vi "HEWH_HeiseBarometer.vi"(8 "error in":errorcluster, 11 "Message Queues out":T1) -> (0 "error out":errorcluster)   [LabVIEW 2023]
uses:
  Tenney/support/Message Queue/All Message Queues.ctl
  Tenney/support/Message Queue/Message Cluster.ctl
  FVIR and LDO/support/Message Queue/Enqueue Message (Single).vi
  FVIR and LDO/support/Message Queue/Message Queue.lvlib
  Tenney/support/Message Queue/Tenney Message Queue.lvlib
panel:
  out "Barometric Pressure (in Hg)":dbl
  out "Debug":string[](array[string])
  in  "Debug":bool
  out "Loop Count":i32
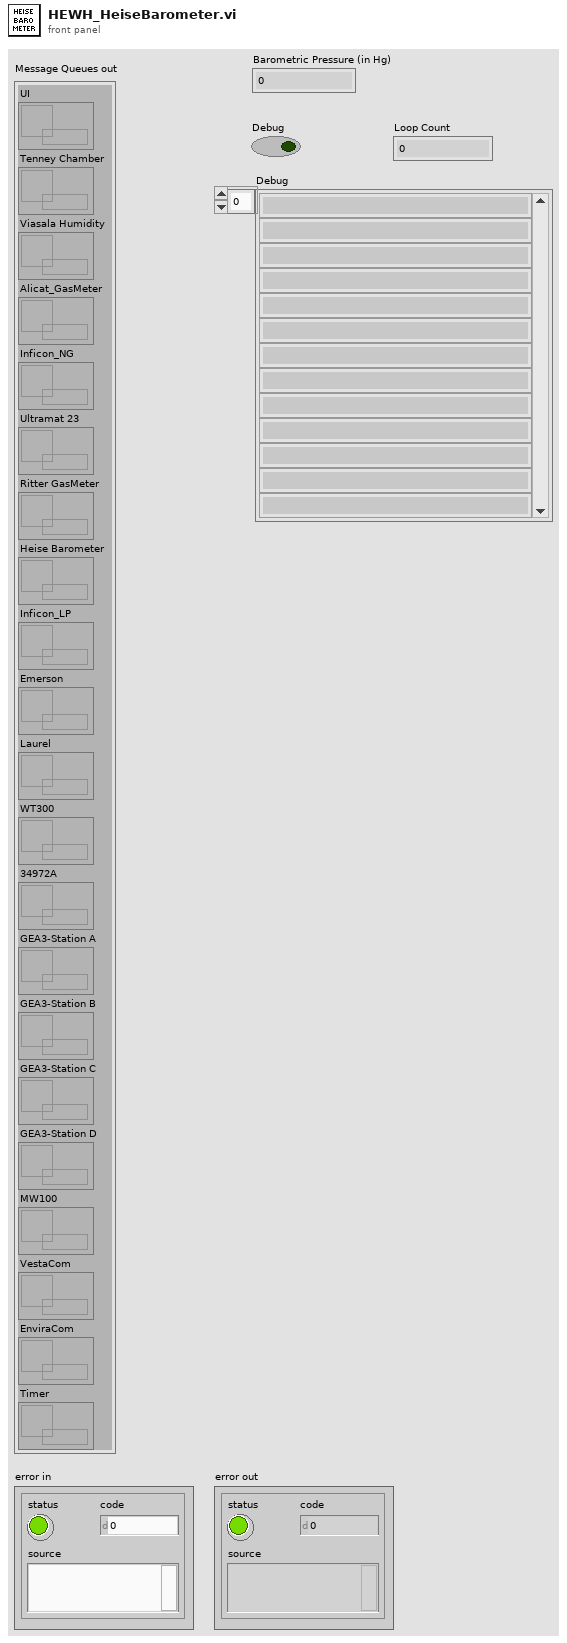
[diagram p1: front panel]
types:
  T1 = typedef "Tenney Message Queue.lvlib/All Message Queues.ctl" = cluster{"UI":refnum<queue>, "Tenney Chamber":refnum<queue>, "Viasala Humidity":refnum<queue>, "Alicat_GasMeter":refnum<queue>, "Inficon_NG":refnum<queue>, "Ultramat 23":refnum<queue>, "Ritter GasMeter":refnum<queue>, "Heise Barometer":refnum<queue>, "Inficon_LP":refnum<queue>, "Emerson":refnum<queue>, "Laurel":refnum<queue>, "WT300":refnum<queue>, "34972A":refnum<queue>, "GEA3-Station A":refnum<queue>, "GEA3-Station B":refnum<queue>, "GEA3-Station C":refnum<queue>, "GEA3-Station D":refnum<queue>, "MW100":refnum<queue>, "VestaCom":refnum<queue>, "EnviraCom":refnum<queue>, "Timer":refnum<queue>}
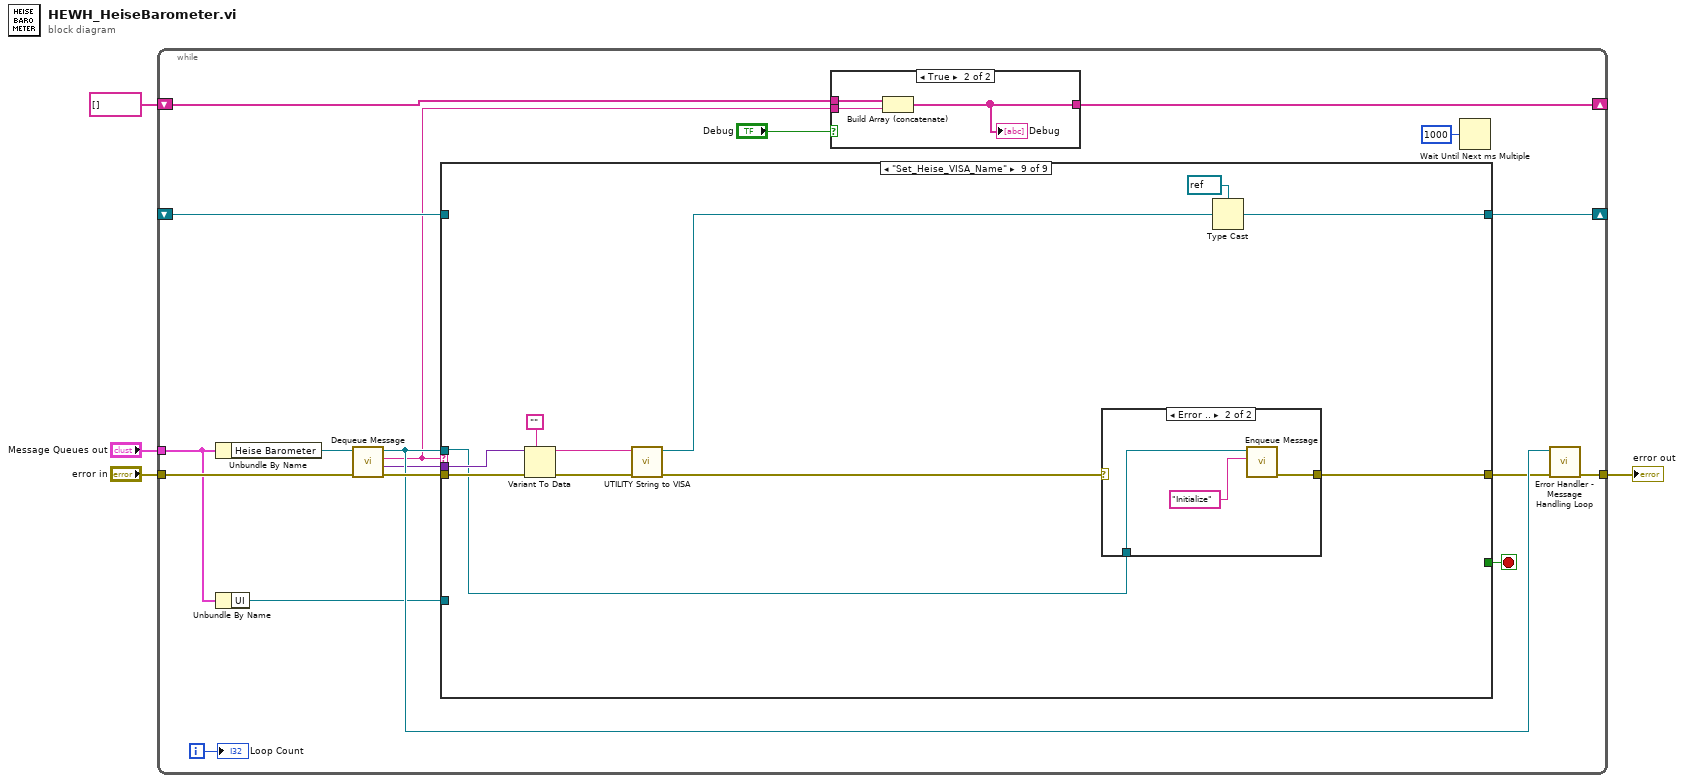
[diagram p0: block diagram]
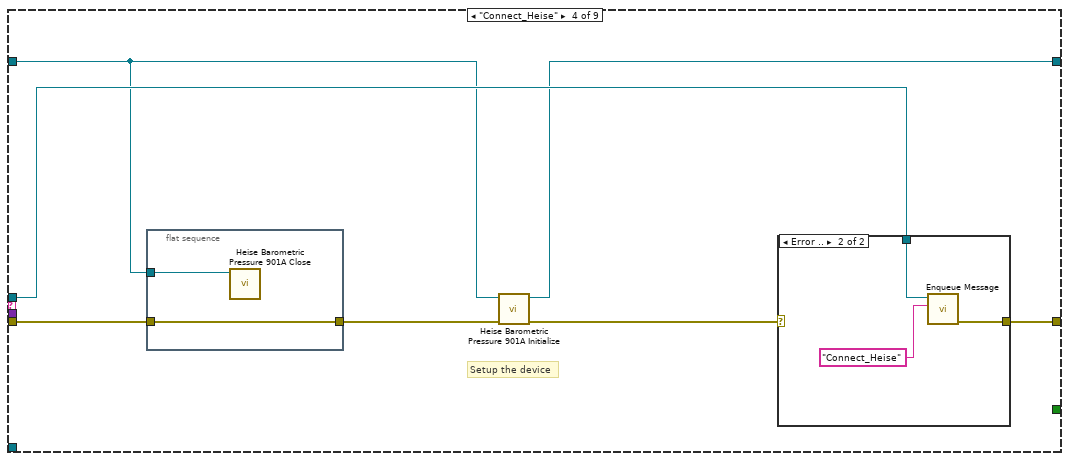
[diagram p6: hidden frame]
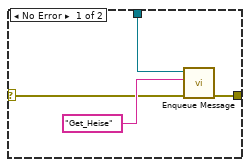
[diagram p7: hidden frame]
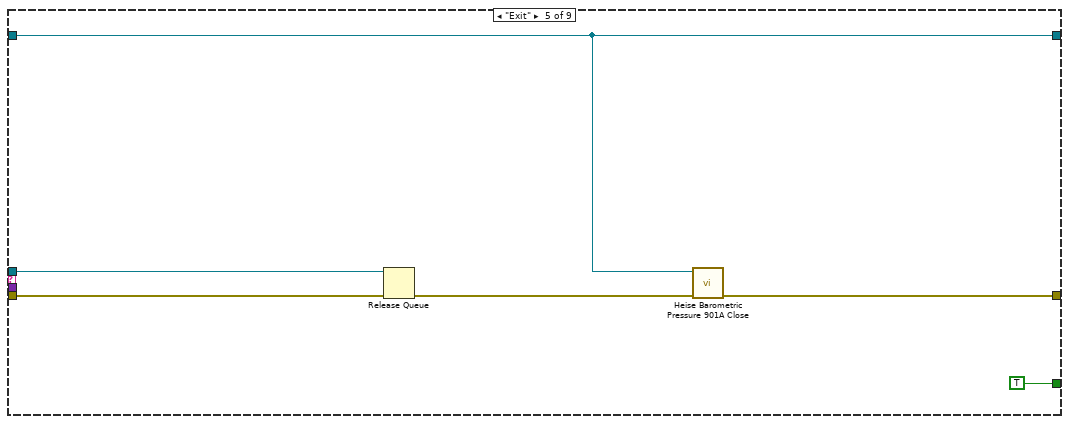
[diagram p8: hidden frame]
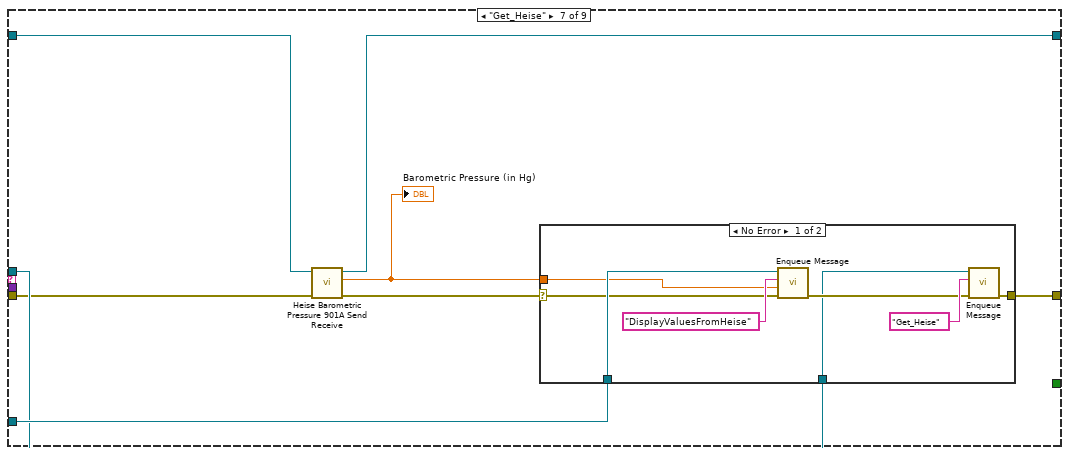
[diagram p10: hidden frame]
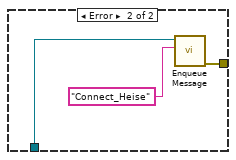
[diagram p11: hidden frame]
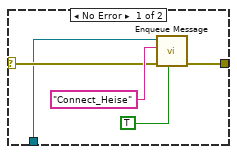
[diagram p13: hidden frame]
diagram:
  n1 = while {
    tunnel: "Message Queues out" -> [w14]
    tunnel: "error in" -> [w21]
    tunnel: [w17] -> w3
    shift-right: [w12] -> _
    shift-left: _ -> [w11]
    shift-right: [w6] -> _
    shift-left: string[] [] -> [w8]
    i -> [w10]
    stop <- w19 stop-if-true
    n2 = Unbundle By Name(w14) -> ("Heise Barometer"=w22:refnum<queue>)
    n3 = Unbundle By Name(w14) -> ("UI"=w13:refnum<queue>)
    n4 = call "Dequeue Message.vi"("error in (no error)"=w21, "Message Queue"=w22) -> ("error out"=w20:errorcluster, "Message Data"=w5:variant, "Message"=w7:string, "dup Message Queue"=w18:refnum<queue>)  [unwired: 6 in]
    n5 = case shown="\"Set_Heise_VISA_Name\"" w7 {
      tunnel: w20 -> [w27 w29 w31 w35 w49 w55 w61 w76 w87]
      tunnel: [w27 w29 w31 w39 w51 w55 w63 w76 w82] -> w16
      tunnel: [_ _ _ _ TRUE _ _ _ _] -> w19
      tunnel: w18 -> [_ _ _ w38 w53 _ w62 _ w81]
      tunnel: w13 -> [_ _ _ _ _ _ w64 _ _]
      tunnel: [w28 w30 w32 w37 w50 w56 w59 w77 w78] -> w12
      tunnel: w11 -> [w28 w30 w32 w34 w50 w56 w60 w77 _]
      tunnel: w5 -> [_ _ _ _ _ _ _ _ w86]
      frame "---------- Setup ----------" {
      }
      frame Default {
      }
      frame "Initialize" {
      }
      frame "Connect_Heise" {
        # "Setup the device"
        n6 = flat-sequence {
          tunnel: w35 -> [w40]
          tunnel: w34 -> [w41]
          tunnel: [w40] -> w33
          frame #0 {
            n7 = call "Heise Barometric Pressure 901A Close.vi"("VISA Refnum in"=w41) -> ()  [unwired: 10 in, 1 out]
          }
        }
        n8 = call "Heise Barometric Pressure 901A Initialize.vi"("error in (no error)"=w33, "VISA Refnum in"=w34) -> ("error out"=w36:errorcluster, "VISA Refnum out"=w37:refnum<visa-resource-name>)  [unwired: 8 in]
        n9 = case shown="Error .." w36 {
          selector: w36 -> [w42 _]
          tunnel: [w44 w47] -> w39
          tunnel: w38 -> [w43 w46]
          frame No Error {
            n10 = call-poly "Enqueue Message.vi"("error in (no error)"=w42, "Message"="Get_Heise", "Message Queue"=w43) -> ("error out"=w44:errorcluster)  [unwired: 7 in, 1 out]
          }
          frame Error {
            n11 = call-poly "Enqueue Message.vi"("Message"="Connect_Heise", "Message Queue"=w46) -> ("error out"=w47:errorcluster)  [unwired: 8 in, 1 out]
          }
        }
      }
      frame "Exit" {
        n12 = Release Queue(queue=w53, error in (no error)=w49) -> (error out=w52:errorcluster)  [unwired: 1 in, 2 out]
        n13 = call "Heise Barometric Pressure 901A Close.vi"("error in (no error)"=w52, "VISA Refnum in"=w50) -> ("error out"=w51:errorcluster)  [unwired: 9 in]
      }
      frame "---------- Data Collection ----------" {
      }
      frame "Get_Heise" {
        n14 = call "Heise Barometric Pressure 901A Send Receive.vi"("error in (no error)"=w61, "VISA Refnum in"=w60) -> ("error out"=w57:errorcluster, "Barometric Pressure (in Hg)"=w58:dbl, "VISA Refnum out"=w59:refnum<visa-resource-name>)  [unwired: 5 in, 2 out]
        "Barometric Pressure (in Hg)" <- w58
        n15 = case shown="No Error" w57 {
          selector: w57 -> [w65 _]
          tunnel: w64 -> [w71 _]
          tunnel: [w68 w74] -> w63
          tunnel: w62 -> [w67 w73]
          tunnel: w58 -> [w66 _]
          frame No Error {
            n16 = call-poly "Enqueue Message.vi"("error in (no error)"=w65, "Message Data"=w66, "Message"="DisplayValuesFromHeise", "Message Queue"=w71) -> ("error out"=w69:errorcluster)  [unwired: 6 in, 1 out]
            n17 = call-poly "Enqueue Message.vi"("error in (no error)"=w69, "Message"="Get_Heise", "Message Queue"=w67) -> ("error out"=w68:errorcluster)  [unwired: 7 in, 1 out]
          }
          frame Error {
            n18 = call-poly "Enqueue Message.vi"("Message"="Connect_Heise", "Message Queue"=w73) -> ("error out"=w74:errorcluster)  [unwired: 8 in, 1 out]
          }
        }
      }
      frame "---------- Events ----------" {
      }
      frame "Set_Heise_VISA_Name" {
        n19 = Variant To Data(error in=w87, type="", Variant=w86) -> (data=w84:string, error out=w85:errorcluster)
        n20 = call "UTILITY String to VISA.vi"("error in (no error)"=w85, "VISA Name"=w84) -> ("error out"=w83:errorcluster, "VISA resource name out"=w80:refnum<visa-resource-name>)  [unwired: 8 in]
        n21 = case shown="Error .." w83 {
          selector: w83 -> [w91 _]
          tunnel: [w90 w95] -> w82
          tunnel: w81 -> [w89 w94]
          frame No Error {
            n22 = call-poly "Enqueue Message.vi"("Priority Message? (F)"=TRUE, "error in (no error)"=w91, "Message"="Connect_Heise", "Message Queue"=w89) -> ("error out"=w90:errorcluster)  [unwired: 6 in, 1 out]
          }
          frame Error {
            n23 = call-poly "Enqueue Message.vi"("Message"="Initialize", "Message Queue"=w94) -> ("error out"=w95:errorcluster)  [unwired: 8 in, 1 out]
          }
        }
        n24 = Type Cast(type=refnum<visa-resource-name> refnum ("VISA resource name out"), x=w80) -> (*(type *) &x=w78:refnum<visa-resource-name>)
      }
    }
    n25 = case shown="True" "Debug" {
      tunnel: w7 -> [_ w26]
      tunnel: w8 -> [w23 w25]
      tunnel: [w23 w24] -> w6
      frame False {
      }
      frame True {
        n26 = Build Array (concatenate)(w25, w26) -> (w24:string[])
        "Debug" <- w24
      }
    }
    n27 = Wait Until Next ms Multiple(millisecond multiple=u32 1000) -> ()  [unwired: 1 out]
    n28 = call "Error Handler - Message Handling Loop.vi"("error in (no error)"=w16, "Message Queue"=w18) -> ("dup error in"=w17:errorcluster)  [unwired: 8 in, 1 out]
    "Loop Count" <- w10
  }
  "error out" <- w3
